vi "Process SDL Events.vi"(11 "Main Controller Actor in":refnum<class "Main Controller Actor.lvclass">) -> (3 "Main Controller Actor out":refnum<class "Main Controller Actor.lvclass">)   [LabVIEW 2021, in "Main Controller Actor.lvclass"]
uses:
  Main Controller Actor.lvclass
  Player.ctl
  LabSDL2/Source/Libraries/LibSDL2 Wrapper/LibSDL2.lvlib
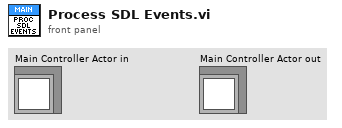
[diagram p1: front panel]
types:
  T1 = typedef "Main Controller Actor.lvclass/Player.ctl" = enum16{"1", "2"}
  T2 = typedef "LibSDL2.lvlib/Keyboard Event.ctl" = cluster{"Type":u32, "Timestamp":u32, "Window ID":u32, "State":u8, "Repeat":u8, "Padding 1":u8, "Padding 2":u8, "Key Sym":cluster{"Scan Code":u32, "Sym":i32, "Mod":u16, "Unused":u32}}
  T3 = typedef "LibSDL2.lvlib/Joysitck Axis Event.ctl" = cluster{"Type":u32, "Timestamp":u32, "Which":i32, "Axis":u8, "Padding 1":u8, "Padding 2":u8, "Padding 3":u8, "Value":i16, "Padding 4":u16}
  T4 = typedef "LibSDL2.lvlib/Joysitck Button Event.ctl" = cluster{"Type":u32, "Timestamp":u32, "Which":i32, "Button":u8, "State":u8, "Padding 1":u8, "Padding 2":u8}
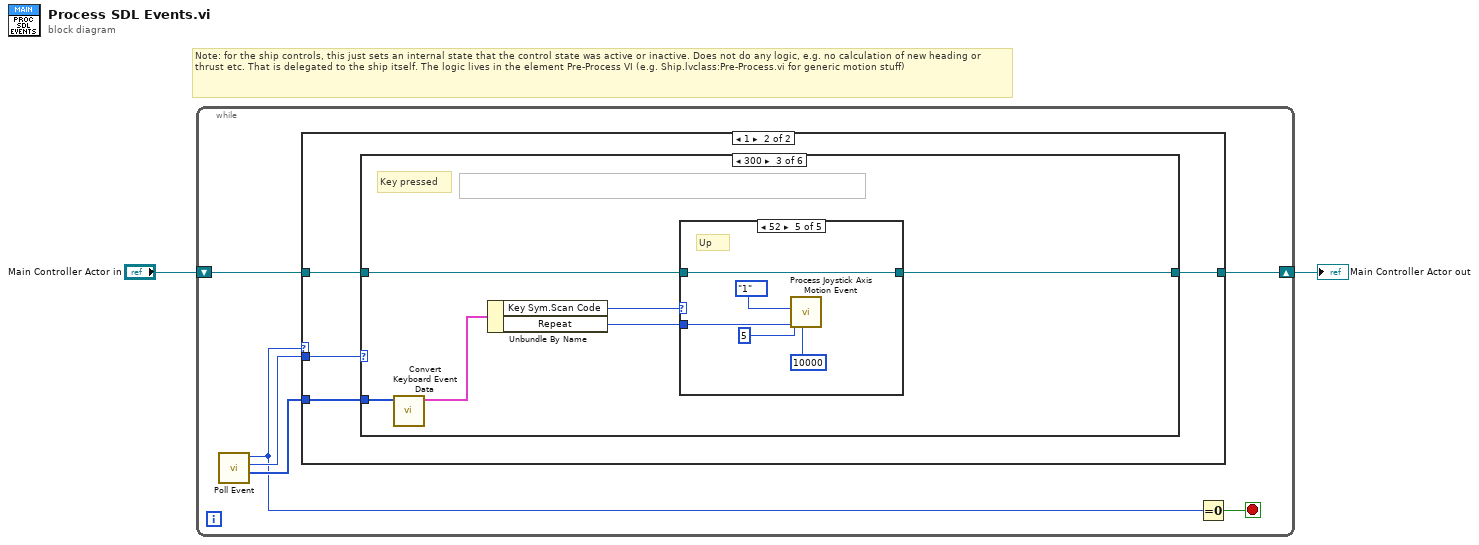
[diagram p0: block diagram]
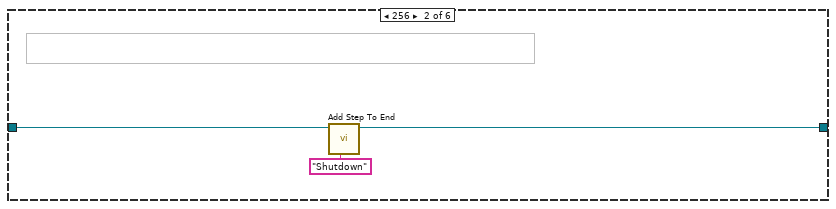
[diagram p4: hidden frame]
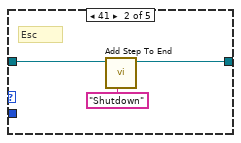
[diagram p6: hidden frame]
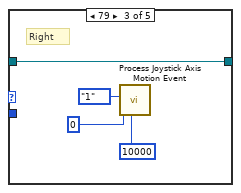
[diagram p7: hidden frame]
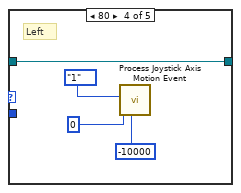
[diagram p8: hidden frame]
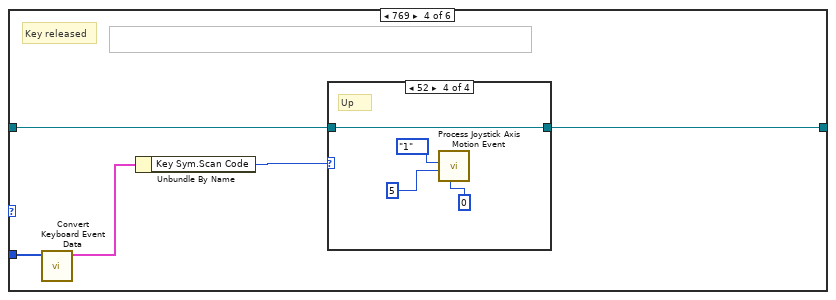
[diagram p9: hidden frame]
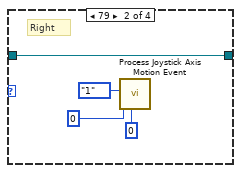
[diagram p11: hidden frame]
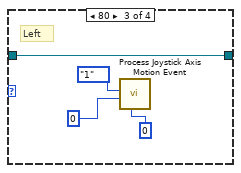
[diagram p12: hidden frame]
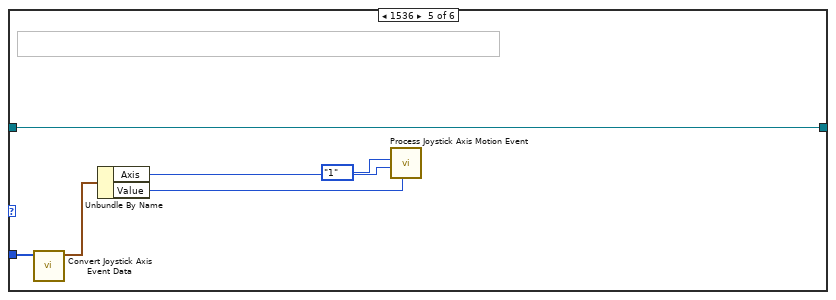
[diagram p13: hidden frame]
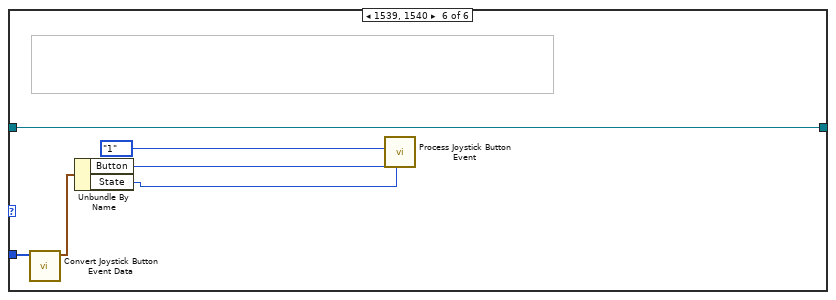
[diagram p14: hidden frame]
diagram:
  # "Note: for the ship controls, this just sets an internal state that the control state was active or inactive. Does not do any logic, e.g. no calculation of new heading or thrust etc. That is delegated to the ship itself. The logic lives in the element Pre-Process VI (e.g. Ship.lvclass:Pre-Process.vi for generic motion stuff)"
  n1 = while {
    shift-right: [w5] -> w2
    shift-left: "Main Controller Actor in" -> [w8]
    stop <- w3 stop-if-true
    n2 = call "Poll Event.vi"() -> ("Event Data"=w7:u8[], "Event Type"=w6:u32, "Return"=w4:i32)  [unwired: 8 in, 1 out]
    n3 = case shown="1" w4 {
      tunnel: w6 -> [_ w13]
      tunnel: w7 -> [_ w10]
      tunnel: w8 -> [w9 w12]
      tunnel: [w9 w11] -> w5
      frame Default {
      }
      frame 1 {
        n4 = case shown="300" w13 {
          tunnel: w12 -> [w14 w17 w23 w45 w59 w65]
          tunnel: [w14 w16 w22 w44 w59 w65] -> w11
          tunnel: w10 -> [_ _ w21 w43 w62 w68]
          frame Default {
          }
          frame 256 {
            n5 = call-dynamic "Add Step To End.vi"("Step Name"="Shutdown", "Actor in"=w17) -> ("Actor out"=w16:refnum<class "Main Controller Actor.lvclass">)  [unwired: 8 in, 1 out]
          }
          frame 768 {
            # "Key pressed"
            n6 = call "Convert Keyboard Event Data.vi"("Event Data"=w21) -> ("Keyboard Event"=w20:T2)  [unwired: 10 in]
            n7 = Unbundle By Name(w20) -> ("Key Sym.Scan Code"=w19:u32, "Repeat"=w18:u8)
            n8 = case shown="52" w19 {
              tunnel: w23 -> [w24 w27 w28 w32 w37]
              tunnel: [w24 w26 w28 w32 w37] -> w22
              tunnel: w18 -> [_ _ _ _ w36]
              frame Default {
              }
              frame 41 {
                # "Esc"
                n9 = call-dynamic "Add Step To End.vi"("Step Name"="Shutdown", "Actor in"=w27) -> ("Actor out"=w26:refnum<class "Main Controller Actor.lvclass">)  [unwired: 8 in, 1 out]
              }
              frame 79 {
                # "Right"
                n10 = call "Process Joystick Axis Motion Event.vi"("Value"=i16 10000, "Axis"=u8 0, "Player"=Player."1") -> ()  [unwired: 9 in]
              }
              frame 80 {
                # "Left"
                n11 = call "Process Joystick Axis Motion Event.vi"("Value"=i16 -10000, "Axis"=u8 0, "Player"=Player."1") -> ()  [unwired: 9 in]
              }
              frame 82 {
                # "Up"
                n12 = call "Process Joystick Axis Motion Event.vi"("Value"=i16 10000, "Repeat"=w36, "Axis"=u8 5, "Player"=Player."1") -> ()  [unwired: 8 in]
              }
            }
          }
          frame 769 {
            # "Key released"
            n13 = call "Convert Keyboard Event Data.vi"("Event Data"=w43) -> ("Keyboard Event"=w42:T2)  [unwired: 10 in]
            n14 = Unbundle By Name(w42) -> ("Key Sym.Scan Code"=w41:u32)
            n15 = case shown="52" w41 {
              tunnel: w45 -> [w46 w47 w51 w55]
              tunnel: [w46 w47 w51 w55] -> w44
              frame 0, Default {
              }
              frame 79 {
                # "Right"
                n16 = call "Process Joystick Axis Motion Event.vi"("Value"=i16 0, "Axis"=u8 0, "Player"=Player."1") -> ()  [unwired: 9 in]
              }
              frame 80 {
                # "Left"
                n17 = call "Process Joystick Axis Motion Event.vi"("Value"=i16 0, "Axis"=u8 0, "Player"=Player."1") -> ()  [unwired: 9 in]
              }
              frame 82 {
                # "Up"
                n18 = call "Process Joystick Axis Motion Event.vi"("Value"=i16 0, "Axis"=u8 5, "Player"=Player."1") -> ()  [unwired: 9 in]
              }
            }
          }
          frame 1536 {
            n19 = call "Convert Joystick Axis Event Data.vi"("Event Data"=w62) -> ("Joystick Axis Event"=w61:T3)  [unwired: 10 in]
            n20 = Unbundle By Name(w61) -> ("Axis"=w64:u8, "Value"=w63:i16)
            n21 = call "Process Joystick Axis Motion Event.vi"("Value"=w63, "Axis"=w64, "Player"=Player."1") -> ()  [unwired: 9 in]
          }
          frame 1539, 1540 {
            n22 = call "Convert Joystick Button Event Data.vi"("Event Data"=w68) -> ("Joystick Button Event"=w67:T4)  [unwired: 10 in]
            n23 = Unbundle By Name(w67) -> ("Button"=w70:u8, "State"=w69:u8)
            n24 = call "Process Joystick Button Event.vi"("State"=w69, "Button"=w70, "Player"=Player."1") -> ()  [unwired: 9 in]
          }
        }
      }
    }
    n25 = Equal To 0?(x=w4) -> (x = 0?=w3:bool)
  }
  "Main Controller Actor out" <- w2
